vi "Init Events.vi"(8 "error in (no error)":errorcluster, 11 "picoG in":refnum<class "picoG.lvclass">) -> (0 "error out":errorcluster, 3 "picoG out":refnum<class "picoG.lvclass">)   [LabVIEW 2020, in "PicoG-App.lvlib" / "picoG.lvclass"]
uses:
  picoG.lvclass
  App Watcher/App Update Data.ctl
  ViaApp/ViaApp.lvclass
  Builds/picoG/ppl/PicoG-Core.lvlibp/PicoG-Processor/PicoG-Core/Platform/Platform.lvclass
  Device/Device.lvclass
  Deploy Data.ctl
  picoG.lvclass/picoG.ctl
  App Watcher/App Watcher.lvclass
  PicoG-App.lvlib
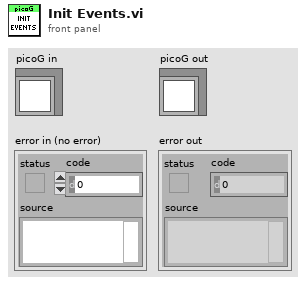
[diagram p1: front panel]
types:
  T1 = typedef "PicoG-App.lvlib/Deploy Data.ctl" = cluster{"App":refnum<class "ViaApp.lvclass">, "Device":refnum<class "Device.lvclass">}
  T2 = typedef "PicoG-App.lvlib/App Watcher.lvclass/App Update Data.ctl" = cluster{"App":refnum<class "ViaApp.lvclass">}
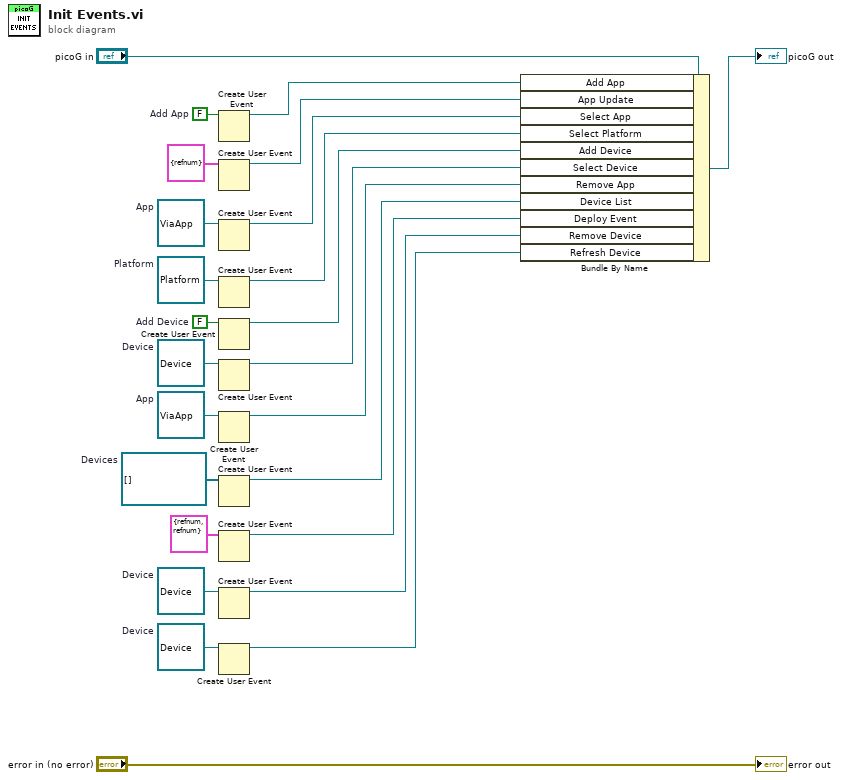
[diagram p0: block diagram]
diagram:
  w2 = refnum<class "Device.lvclass"> refnum  # Device
  w4 = refnum<class "Device.lvclass"> refnum  # Device
  w8 = refnum<class "Device.lvclass">[] []  # Devices
  w10 = refnum<class "ViaApp.lvclass"> refnum  # App
  w12 = refnum<class "Device.lvclass"> refnum  # Device
  w14 = FALSE  # Add Device
  w16 = refnum<class "Platform.lvclass"> refnum  # Platform
  w18 = refnum<class "ViaApp.lvclass"> refnum  # App
  w22 = FALSE  # Add App
  n1 = Create User Event(user event datatype=w22) -> (user event=w21:refnum<user-event>)  [unwired: 1 in, 1 out]
  n2 = Create User Event(user event datatype=T2 {"App"=refnum} ("App Update Data")) -> (user event=w19:refnum<user-event>)  [unwired: 1 in, 1 out]
  n3 = Create User Event(user event datatype=w18) -> (user event=w17:refnum<user-event>)  [unwired: 1 in, 1 out]
  n4 = Create User Event(user event datatype=w16) -> (user event=w15:refnum<user-event>)  [unwired: 1 in, 1 out]
  n5 = Create User Event(user event datatype=w14) -> (user event=w13:refnum<user-event>)  [unwired: 1 in, 1 out]
  n6 = Create User Event(user event datatype=w12) -> (user event=w11:refnum<user-event>)  [unwired: 1 in, 1 out]
  n7 = Create User Event(user event datatype=w10) -> (user event=w9:refnum<user-event>)  [unwired: 1 in, 1 out]
  n8 = Create User Event(user event datatype=w8) -> (user event=w7:refnum<user-event>)  [unwired: 1 in, 1 out]
  n9 = Create User Event(user event datatype=T1 {"App"=refnum, "Device"=refnum} ("Deploy Data")) -> (user event=w5:refnum<user-event>)  [unwired: 1 in, 1 out]
  n10 = Create User Event(user event datatype=w4) -> (user event=w3:refnum<user-event>)  [unwired: 1 in, 1 out]
  n11 = Create User Event(user event datatype=w2) -> (user event=w1:refnum<user-event>)  [unwired: 1 in, 1 out]
  n12 = Bundle By Name(cluster="picoG in", "Add App"=w21, "App Update"=w19, "Select App"=w17, "Select Platform"=w15, "Add Device"=w13, "Select Device"=w11, "Remove App"=w9, "Device List"=w7, "Deploy Event"=w5, "Remove Device"=w3, "Refresh Device"=w1) -> (→"picoG out":refnum<class "picoG.lvclass">)
  "error out" <- "error in (no error)"
